vi "Target Detection.vi"(5 "Left Cam?":bool, 6 "Vision Mode":T1 caption="Vision Mode (Reported by Robot)", 7 "Score Cutoff":dbl(slide)=54.248366013071895 scale=0.0..100.0, 9 "HSV Filter":T2, 10 "Src Image":T5) -> (0 "Vision Targets":T4, 2 "Annotated Image":T5, 3 "Mask":T5)   [LabVIEW 2013]
uses:
  <vilib>/vision/Image Controls.llb/IMAQ Image.ctl
  Common Code/Goal Info.ctl
  Common Code/Vision Mode.ctl
panel:
  out "Mask Display":T5(plugin-control)
  in  "Area Size Limit %":dbl=0.06 format="%#_13g"
  out "Color Components":T6={"Hue"={110.0, 142.0}, "Sat"={138.0, 255.0}, "Val"={139.0, 198.0}} {"Val" scale=0.0..255.0; "Sat" scale=0.0..255.0; "Hue" scale=0.0..255.0 scale format="%#_3g"}
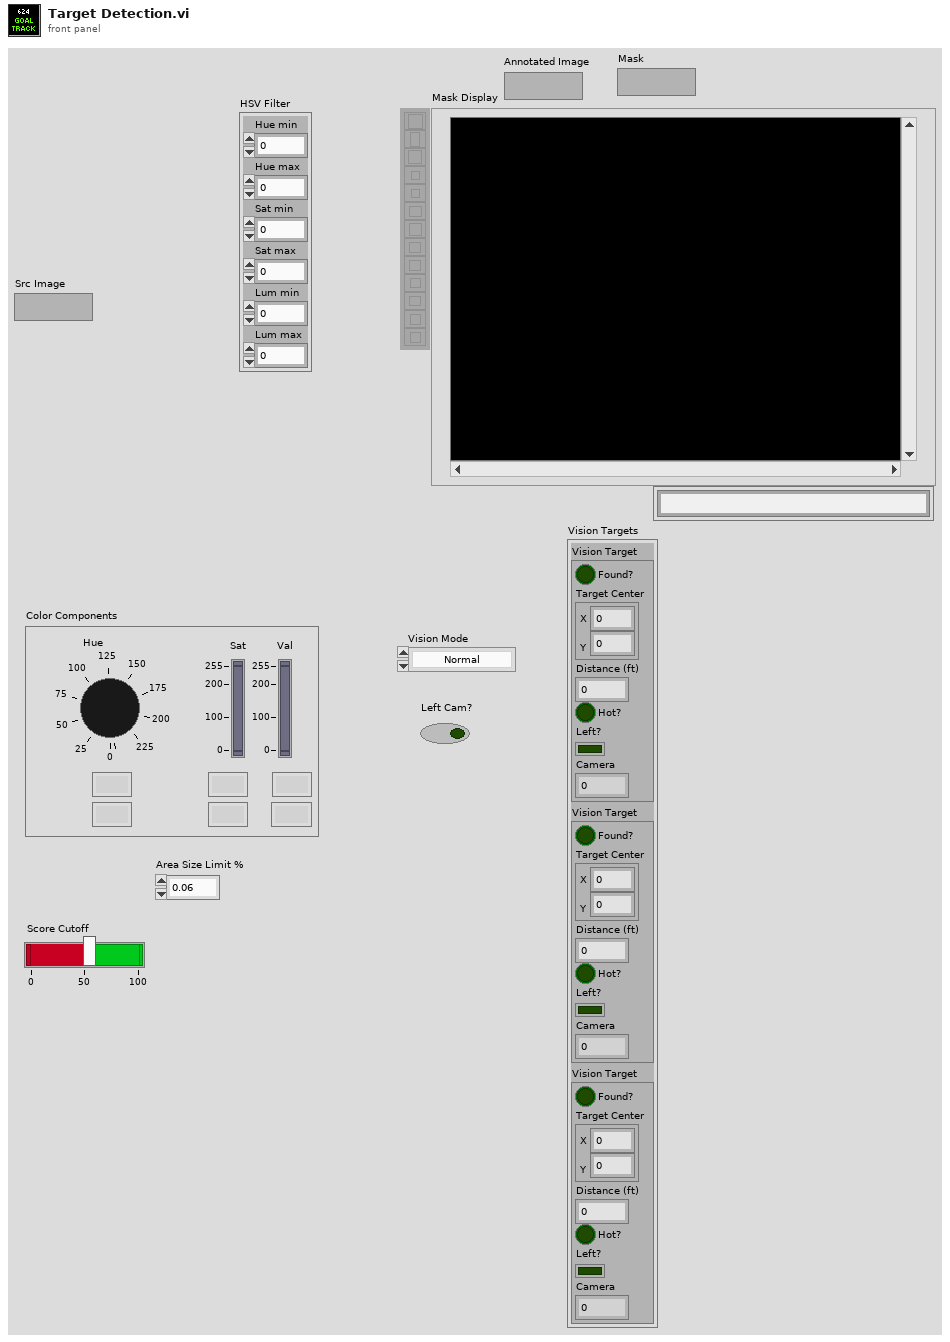
[diagram p1: front panel]
types:
  T1 = typedef "Vision Mode.ctl" = enum16{"Normal", "Extreme Left", "Extreme Right"}
  T2 = cluster{"Hue min":dbl, "Hue max":dbl, "Sat min":dbl, "Sat max":dbl, "Lum min":dbl, "Lum max":dbl}
  T3 = typedef "Goal Info.ctl" = cluster{"Found?":bool, "Target Center":cluster{"X":dbl, "Y":dbl}, "Distance (ft)":dbl, "Hot?":bool, "Left?":bool, "Camera":i16}
  T4 = cluster{"Vision Target":T3, "Vision Target":T3, "Vision Target":T3}
  T5 = typedef "IMAQ Image.ctl" = refnum<image>
  T6 = cluster{"Hue":cluster{dbl, dbl}, "Sat":cluster{dbl, dbl}, "Val":cluster{dbl, dbl}}
  T7 = cluster{"Horizontal":bool, "Aspect Score":dbl, "Rect Score":dbl, cluster{"Left":dbl, "Top":dbl, "Right":dbl, "Bottom":dbl}, "Equiv H":dbl, "Equiv V":dbl}[]
  T8 = typedef "TargetType.ctl" = enum16{"Not Hot", "Hot"}
  T9 = cluster{"Scores":cluster{"Total":dbl, "Left":dbl, "Right":dbl, "Ratio":dbl, "Vertical":dbl, "index":i32, "State":T8}, "Verticals":cluster{"Horizontal?":bool, "Aspect Score":dbl, "Rect Score":dbl, cluster{"Left":dbl, "Top":dbl, "Right":dbl, "Bottom":dbl}, "Equiv H":dbl, "Equiv V":dbl}, "Horizontals":cluster{"Horizontal?":bool, "Aspect Score":dbl, "Rect Score":dbl, cluster{"Left":dbl, "Top":dbl, "Right":dbl, "Bottom":dbl}, "Equiv H":dbl, "Equiv V":dbl}, "Validated":bool}[]
  T10 = cluster{"Distance (ft)":dbl, "Target Center (-1 to 1)":cluster{"X":dbl, "Y":dbl}, "Left":bool, "State":T8}[]
  T11 = cluster{"Scores":cluster{"Total":dbl, "Left":dbl, "Right":dbl, "Ratio":dbl, "Vertical":dbl, "index":i32, "State":T8}, "Verticals":cluster{"Horizontal?":bool, "Aspect Score":dbl, "Rect Score":dbl, cluster{"Left":dbl, "Top":dbl, "Right":dbl, "Bottom":dbl}, "Equiv H":dbl, "Equiv V":dbl}, "Horizontals":cluster{"Horizontal?":bool, "Aspect Score":dbl, "Rect Score":dbl, cluster{"Left":dbl, "Top":dbl, "Right":dbl, "Bottom":dbl}, "Equiv H":dbl, "Equiv V":dbl}, "Distance (ft)":dbl, "Target Center (-1 to 1)":cluster{"X":dbl, "Y":dbl}}[]
  T12 = cluster{cluster{"Scores":cluster{"Total":dbl, "Left":dbl, "Right":dbl, "Ratio":dbl, "Vertical":dbl, "index":i32, "State":T8}, "Verticals":cluster{"Horizontal?":bool, "Aspect Score":dbl, "Rect Score":dbl, cluster{"Left":dbl, "Top":dbl, "Right":dbl, "Bottom":dbl}, "Equiv H":dbl, "Equiv V":dbl}, "Horizontals":cluster{"Horizontal?":bool, "Aspect Score":dbl, "Rect Score":dbl, cluster{"Left":dbl, "Top":dbl, "Right":dbl, "Bottom":dbl}, "Equiv H":dbl, "Equiv V":dbl}, "Distance (ft)":dbl, "Target Center (-1 to 1)":cluster{"X":dbl, "Y":dbl}}, cluster{"Distance (ft)":dbl, "Target Center (-1 to 1)":cluster{"X":dbl, "Y":dbl}, "Left":bool, "State":T8}}[]
  T13 = cluster{"Distance (ft)":dbl, "Target Center (-1 to 1)":cluster{"X":dbl, "Y":dbl}, "Left":bool, "State":T8}
  T14 = cluster{cluster{"Scores":cluster{"Total":dbl, "Left":dbl, "Right":dbl, "Ratio":dbl, "Vertical":dbl, "index":i32, "State":T8}, "Verticals":cluster{"Horizontal?":bool, "Aspect Score":dbl, "Rect Score":dbl, cluster{"Left":dbl, "Top":dbl, "Right":dbl, "Bottom":dbl}, "Equiv H":dbl, "Equiv V":dbl}, "Horizontals":cluster{"Horizontal?":bool, "Aspect Score":dbl, "Rect Score":dbl, cluster{"Left":dbl, "Top":dbl, "Right":dbl, "Bottom":dbl}, "Equiv H":dbl, "Equiv V":dbl}, "Distance (ft)":dbl, "Target Center (-1 to 1)":cluster{"X":dbl, "Y":dbl}}, cluster{"Distance (ft)":dbl, "Target Center (-1 to 1)":cluster{"X":dbl, "Y":dbl}, "Left":bool, "State":T8}}
  T15 = cluster{"Scores":cluster{"Total":dbl, "Left":dbl, "Right":dbl, "Ratio":dbl, "Vertical":dbl, "index":i32, "State":T8}, "Verticals":cluster{"Horizontal?":bool, "Aspect Score":dbl, "Rect Score":dbl, cluster{"Left":dbl, "Top":dbl, "Right":dbl, "Bottom":dbl}, "Equiv H":dbl, "Equiv V":dbl}, "Horizontals":cluster{"Horizontal?":bool, "Aspect Score":dbl, "Rect Score":dbl, cluster{"Left":dbl, "Top":dbl, "Right":dbl, "Bottom":dbl}, "Equiv H":dbl, "Equiv V":dbl}, "Distance (ft)":dbl, "Target Center (-1 to 1)":cluster{"X":dbl, "Y":dbl}}
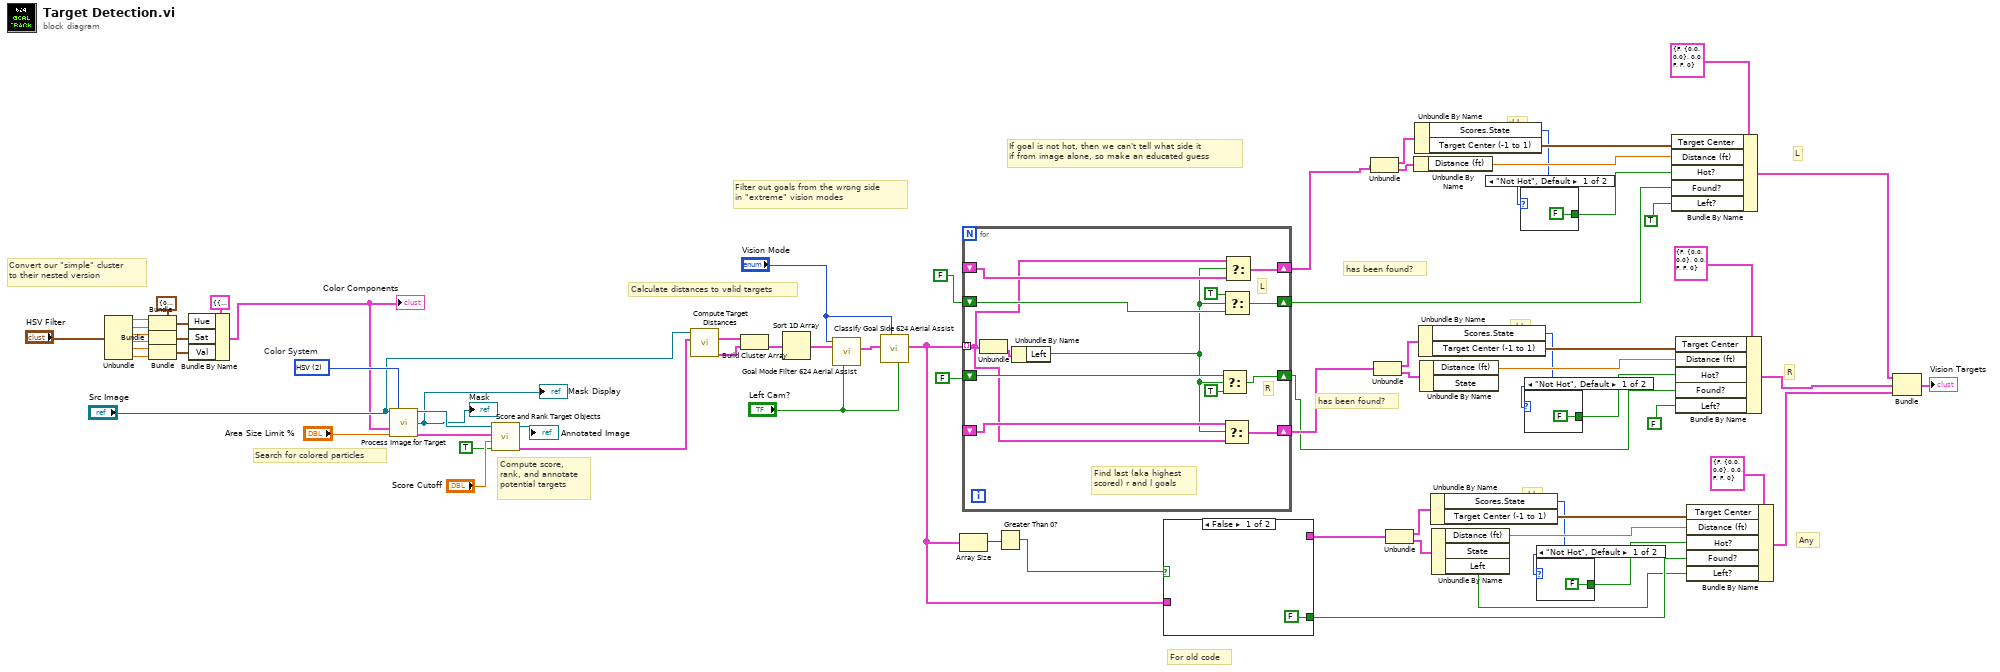
[diagram p0: block diagram]
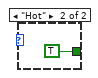
[diagram p2: hidden frame]
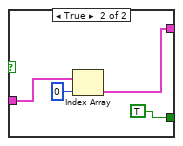
[diagram p3: hidden frame]
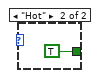
[diagram p4: hidden frame]
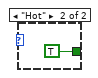
[diagram p5: hidden frame]
diagram:
  w19 = cluster{dbl, dbl} {0.0, 0.0} ("Hue")
  w64 = u16 2 items=["RGB", "HSL", "HSV", "HSI"]  # Color System
  # "has been found?"
  # "has been found?"
  # "Filter out goals from the wrong side\nin \"extreme\" vision modes"
  # "If goal is not hot, then we can't tell what side it\nif from image alone, so make an educated guess"
  # "Convert our \"simple\" cluster\nto their nested version"
  # "Calculate distances to valid targets"
  # "Any"
  # "tlrb"
  # "For old code"
  # "R"
  # "L"
  # "tlrb"
  # "tlrb"
  # "Search for colored particles"
  # "Compute score,\nrank, and annotate\npotential targets"
  n1 = Unbundle("HSV Filter") -> ("Hue min"=w16:dbl, "Hue max"=w15:dbl, "Sat min"=w14:dbl, "Sat max"=w13:dbl, "Lum min"=w12:dbl, "Lum max"=w11:dbl)
  n2 = Bundle(cluster=w19, w16, w15) -> (w20:cluster{dbl, dbl})
  n3 = Bundle(cluster=w19, w14, w13) -> (w18:cluster{dbl, dbl})
  n4 = Bundle(cluster=w19, w12, w11) -> (w17:cluster{dbl, dbl})
  n5 = Bundle By Name(cluster=T6 {"Hue"={104.99307782068851, 142.0}, "Sat"={138.0, 255.0}, "Val"={139.0, 198.0}} ("Color Components"), "Hue"=w20, "Sat"=w18, "Val"=w17) -> (w21:T6)
  "Color Components" <- w21
  n6 = call "Process Image for Target.vi"("Src Image"="Src Image", "Color Mode"=w64, "Color Components"=w21, "Area Cutoff %"="Area Size Limit %") -> ("Src Image Out"=w68:T5, "Threshold"=→"Mask Display" →"Mask":T5, "Particles"=w65:T7)  [unwired: 9 in]
  n7 = call "Score and Rank Target Objects.vi"("Annotate"=TRUE, "Score Limit"="Score Cutoff", "Particles"=w65, "Image in"=w68) -> ("Target Info"=w62:T9, "Annotated Image"=→"Annotated Image":T5)  [unwired: 6 in]
  n8 = call "Compute Target Distances.vi"("Target Info"=w62, "Image in"="Src Image") -> ("Distances"=w58:T10, "Target Info"=w59:T11)  [unwired: 7 in, 1 out]
  n9 = Build Cluster Array(w59, w58) -> (w57:T12)
  n10 = Sort 1D Array(array=w57) -> (sorted array=w8:T12)
  n11 = call "Goal Mode Filter 624 Aerial Assist.vi"("Left Cam?"="Left Cam?", "Targets In"=w8, "Vision Mode"="Vision Mode") -> ("Targets Out"=w7:T12)  [unwired: 7 in]
  n12 = call "Classify Goal Side 624 Aerial Assist.vi"("Left Cam?"="Left Cam?", "Vision Mode"="Vision Mode", "Targets in"=w7) -> ("Targets out"=w6:T12)  [unwired: 8 in]
  n13 = Array Size(array=w6) -> (size(s)=w36:i32)
  n14 = for {
    tunnel: w6 -> [w71] mode=indexing
    shift-right: [w80] -> w53
    shift-left: FALSE -> [w82]
    shift-right: [w75] -> w37
    shift-left: FALSE -> [w76]
    shift-right: [w79] -> w51
    shift-left: _ -> [w78]
    shift-right: [w73] -> w38
    shift-left: _ -> [w72]
    # "Find last (aka highest\nscored) r and l goals"
    # "R"
    # "L"
    n15 = Unbundle(w71) -> (w74:T13)  [unwired: 1 out]
    n16 = Unbundle By Name(w74) -> ("Left"=w70:bool)
    n17 = Select(t=w76, s=w70, f=TRUE ("t")) -> (s? t:f=w75:bool)
    n18 = Select(t=w72, s=w70, f=w71) -> (s? t:f=w73:T14)
    n19 = Select(t=TRUE, s=w70, f=w82) -> (s? t:f=w80:bool)
    n20 = Select(t=w71, s=w70, f=w78) -> (s? t:f=w79:T14)
  }
  n21 = Greater Than 0?(x=w36) -> (x > 0?=w35:bool)
  n22 = case shown="False" w35 {
    tunnel: w6 -> [_ w87]
    tunnel: [_ w85] -> w28
    tunnel: [FALSE TRUE] -> w27
    frame False {
    }
    frame True {
      n23 = Index Array(array=w87, index=0) -> (element=w85:T14)
    }
  }
  n24 = Unbundle(w51) -> (w50:T15, w49:T13)
  n25 = Unbundle(w38) -> (w41:T15, w42:T13)
  n26 = Unbundle(w28) -> (w33:T15, w32:T13)
  n27 = Unbundle By Name(w49) -> ("Distance (ft)"=w48:dbl)
  n28 = Unbundle By Name(w50) -> ("Scores.State"=w3:T8, "Target Center (-1 to 1)"=w47:cluster{"X":dbl, "Y":dbl})
  n29 = Unbundle By Name(w41) -> ("Scores.State"=w2:T8, "Target Center (-1 to 1)"=w44:cluster{"X":dbl, "Y":dbl})
  n30 = Unbundle By Name(w42) -> ("Distance (ft)"=w43:dbl)  [unwired: 1 out]
  n31 = Unbundle By Name(w33) -> ("Scores.State"=w1:T8, "Target Center (-1 to 1)"=w30:cluster{"X":dbl, "Y":dbl})
  n32 = Unbundle By Name(w32) -> ("Distance (ft)"=w31:dbl, "Left"=w26:bool)  [unwired: 1 out]
  n33 = case shown="\"Not Hot\", Default" w3 {
    tunnel: [FALSE TRUE] -> w54
    frame "Not Hot", Default {
    }
    frame "Hot" {
    }
  }
  n34 = case shown="\"Not Hot\", Default" w2 {
    tunnel: [FALSE TRUE] -> w39
    frame "Not Hot", Default {
    }
    frame "Hot" {
    }
  }
  n35 = case shown="\"Not Hot\", Default" w1 {
    tunnel: [FALSE TRUE] -> w34
    frame "Not Hot", Default {
    }
    frame "Hot" {
    }
  }
  n36 = Bundle By Name(cluster=T3 {"Found?"=FALSE, "Target Center"={"X"=0.0, "Y"=0.0}, "Distance (ft)"=0.0, "Hot?"=FALSE, "Left?"=FALSE, "Camera"=0} ("Vision Target"), "Target Center"=w47, "Distance (ft)"=w48, "Hot?"=w54, "Found?"=w53, "Left?"=TRUE) -> (w25:T3)
  n37 = Bundle By Name(cluster=T3 {"Found?"=FALSE, "Target Center"={"X"=0.0, "Y"=0.0}, "Distance (ft)"=0.0, "Hot?"=FALSE, "Left?"=FALSE, "Camera"=0} ("Vision Target"), "Target Center"=w44, "Distance (ft)"=w43, "Hot?"=w39, "Found?"=w37, "Left?"=FALSE) -> (w24:T3)
  n38 = Bundle By Name(cluster=T3 {"Found?"=FALSE, "Target Center"={"X"=0.0, "Y"=0.0}, "Distance (ft)"=0.0, "Hot?"=FALSE, "Left?"=FALSE, "Camera"=0} ("Vision Target"), "Target Center"=w30, "Distance (ft)"=w31, "Hot?"=w34, "Found?"=w27, "Left?"=w26) -> (w23:T3)
  n39 = Bundle("Vision Target"=w25, "Vision Target"=w24, "Vision Target"=w23) -> (→"Vision Targets":T4)  [unwired: 1 in]
